vi "UpdateRequestRaw.vi"(7 "Data to update":T1, 8 "error in":errorcluster, 9 "data":variant, 10 "RequestID":u32) -> (0 "error out":errorcluster)   [LabVIEW 2015, in "DatabaseApi.lvlib"]
uses:
  DatabaseApi.lvlib
  TypeDef/Request/RequestsTableColumnNamesRing.ctl
  TypeDef/Request/RequestsTableDbTableName.ctl
  <vilib>/addons/database/Connection.llb/DB Tools Open Connec (Path).vi
  <vilib>/addons/database/NI_Database_API.lvlib
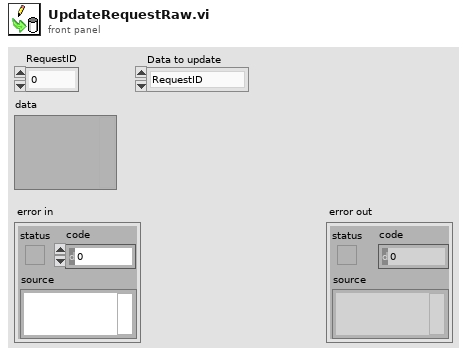
[diagram p1: front panel]
types:
  T1 = typedef "DatabaseApi.lvlib/RequestsTableColumnNamesRing.ctl" = enum16{"RequestID", "PersonnelType", "StartTime", "StartName", "AckTime", "AckName", "FulfilledTime", "FulfilledName", "Description"}
  T2 = typedef "DatabaseApi.lvlib/RequestsTableDbTableName.ctl" = string
  T3 = typedef "NI_Database_API.lvlib/Conn ObjectReference.ctl" = refnum<k1>
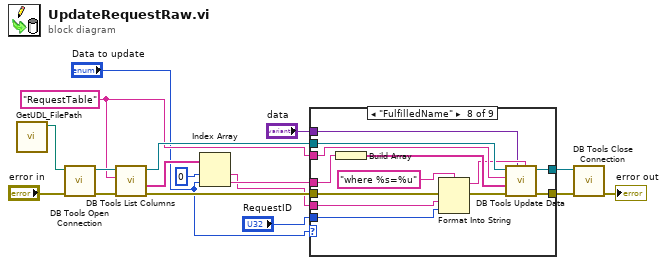
[diagram p0: block diagram]
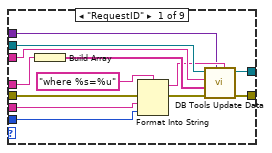
[diagram p2: hidden frame]
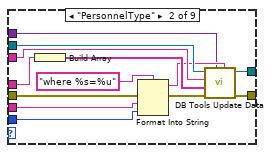
[diagram p3: hidden frame]
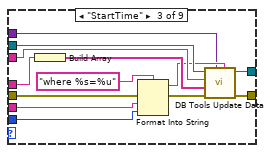
[diagram p4: hidden frame]
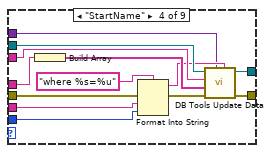
[diagram p5: hidden frame]
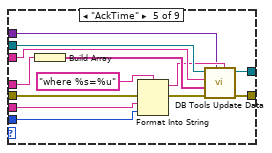
[diagram p6: hidden frame]
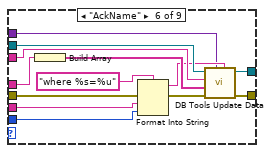
[diagram p7: hidden frame]
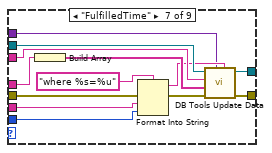
[diagram p8: hidden frame]
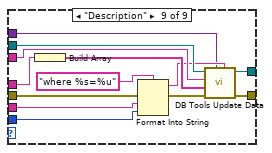
[diagram p9: hidden frame]
diagram:
  w7 = T2 "RequestTable" ("table")
  n1 = call "GetUDL_FilePath.vi"() -> ("UDL file path"=w17:path)  [unwired: 11 in]
  n2 = call-poly <vilib>:"DB Tools Open Connection.vi"("error in (no error)"="error in", "connection information"=w17) -> ("error out"=w14:errorcluster, "connection reference"=w10:T3)  [unwired: 6 in]
  n3 = call <vilib>:"DB Tools List Columns.vi"("error in (no error)"=w14, "table"=w7, "connection reference"=w10) -> ("error out"=w11:errorcluster, "columns"=w8:string[], "connection reference out"=w9:T3)  [unwired: 1 in, 1 out]
  n4 = Index Array(array=w8, index #1=0 ("index"), index #2="Data to update") -> (element #1=w3:string, element #2=w6:string)
  n5 = case shown="\"FulfilledName\"" "Data to update" {
    tunnel: [w30 w43 w56 w69 w82 w95 w108 w121 w134] -> w13
    tunnel: [w29 w42 w55 w68 w81 w94 w107 w120 w133] -> w12
    tunnel: w11 -> [w23 w36 w49 w62 w75 w88 w101 w114 w127]
    tunnel: w9 -> [w28 w41 w54 w67 w80 w93 w106 w119 w132]
    tunnel: w6 -> [w26 w39 w52 w65 w78 w91 w104 w117 w130]
    tunnel: w7 -> [w27 w40 w53 w66 w79 w92 w105 w118 w131]
    tunnel: w3 -> [w21 w34 w47 w60 w73 w86 w99 w112 w125]
    tunnel: "RequestID" -> [w20 w33 w46 w59 w72 w85 w98 w111 w124]
    tunnel: "data" -> [w18 w31 w44 w57 w70 w83 w96 w109 w122]
    frame "RequestID" {
      n6 = Build Array(w26) -> (w25:string[])
      n7 = Format Into String(format string="where %s=%u", error in=w23, w21, w20) -> (resulting string=w19:string, error out=w22:errorcluster)  [unwired: 1 in]
      n8 = call <vilib>:"DB Tools Update Data.vi"("condition"=w19, "data"=w18, "error in (no error)"=w22, "columns"=w25, "table"=w27, "connection reference"=w28) -> ("error out"=w30:errorcluster, "connection reference out"=w29:T3)  [unwired: 4 in]
    }
    frame "PersonnelType" {
      n9 = Build Array(w39) -> (w38:string[])
      n10 = Format Into String(format string="where %s=%u", error in=w36, w34, w33) -> (resulting string=w32:string, error out=w35:errorcluster)  [unwired: 1 in]
      n11 = call <vilib>:"DB Tools Update Data.vi"("condition"=w32, "data"=w31, "error in (no error)"=w35, "columns"=w38, "table"=w40, "connection reference"=w41) -> ("error out"=w43:errorcluster, "connection reference out"=w42:T3)  [unwired: 4 in]
    }
    frame "StartTime" {
      n12 = Build Array(w52) -> (w51:string[])
      n13 = Format Into String(format string="where %s=%u", error in=w49, w47, w46) -> (resulting string=w45:string, error out=w48:errorcluster)  [unwired: 1 in]
      n14 = call <vilib>:"DB Tools Update Data.vi"("condition"=w45, "data"=w44, "error in (no error)"=w48, "columns"=w51, "table"=w53, "connection reference"=w54) -> ("error out"=w56:errorcluster, "connection reference out"=w55:T3)  [unwired: 4 in]
    }
    frame "StartName" {
      n15 = Build Array(w65) -> (w64:string[])
      n16 = Format Into String(format string="where %s=%u", error in=w62, w60, w59) -> (resulting string=w58:string, error out=w61:errorcluster)  [unwired: 1 in]
      n17 = call <vilib>:"DB Tools Update Data.vi"("condition"=w58, "data"=w57, "error in (no error)"=w61, "columns"=w64, "table"=w66, "connection reference"=w67) -> ("error out"=w69:errorcluster, "connection reference out"=w68:T3)  [unwired: 4 in]
    }
    frame "AckTime" {
      n18 = Build Array(w78) -> (w77:string[])
      n19 = Format Into String(format string="where %s=%u", error in=w75, w73, w72) -> (resulting string=w71:string, error out=w74:errorcluster)  [unwired: 1 in]
      n20 = call <vilib>:"DB Tools Update Data.vi"("condition"=w71, "data"=w70, "error in (no error)"=w74, "columns"=w77, "table"=w79, "connection reference"=w80) -> ("error out"=w82:errorcluster, "connection reference out"=w81:T3)  [unwired: 4 in]
    }
    frame "AckName" {
      n21 = Build Array(w91) -> (w90:string[])
      n22 = Format Into String(format string="where %s=%u", error in=w88, w86, w85) -> (resulting string=w84:string, error out=w87:errorcluster)  [unwired: 1 in]
      n23 = call <vilib>:"DB Tools Update Data.vi"("condition"=w84, "data"=w83, "error in (no error)"=w87, "columns"=w90, "table"=w92, "connection reference"=w93) -> ("error out"=w95:errorcluster, "connection reference out"=w94:T3)  [unwired: 4 in]
    }
    frame "FulfilledTime" {
      n24 = Build Array(w104) -> (w103:string[])
      n25 = Format Into String(format string="where %s=%u", error in=w101, w99, w98) -> (resulting string=w97:string, error out=w100:errorcluster)  [unwired: 1 in]
      n26 = call <vilib>:"DB Tools Update Data.vi"("condition"=w97, "data"=w96, "error in (no error)"=w100, "columns"=w103, "table"=w105, "connection reference"=w106) -> ("error out"=w108:errorcluster, "connection reference out"=w107:T3)  [unwired: 4 in]
    }
    frame "FulfilledName" {
      n27 = Build Array(w117) -> (w116:string[])
      n28 = Format Into String(format string="where %s=%u", error in=w114, w112, w111) -> (resulting string=w110:string, error out=w113:errorcluster)  [unwired: 1 in]
      n29 = call <vilib>:"DB Tools Update Data.vi"("condition"=w110, "data"=w109, "error in (no error)"=w113, "columns"=w116, "table"=w118, "connection reference"=w119) -> ("error out"=w121:errorcluster, "connection reference out"=w120:T3)  [unwired: 4 in]
    }
    frame "Description" {
      n30 = Build Array(w130) -> (w129:string[])
      n31 = Format Into String(format string="where %s=%u", error in=w127, w125, w124) -> (resulting string=w123:string, error out=w126:errorcluster)  [unwired: 1 in]
      n32 = call <vilib>:"DB Tools Update Data.vi"("condition"=w123, "data"=w122, "error in (no error)"=w126, "columns"=w129, "table"=w131, "connection reference"=w132) -> ("error out"=w134:errorcluster, "connection reference out"=w133:T3)  [unwired: 4 in]
    }
  }
  n33 = call <vilib>:"DB Tools Close Connection.vi"("error in (no error)"=w13, "connection reference"=w12) -> ("error out"=→"error out":errorcluster)  [unwired: 5 in]
